vi "Helper SubVI - Filtered Square Wave.vi"(5 "offset":dbl, 7 "reset signal":bool, 9 "duty cycle (%)":dbl=50.0 format="%#.6g", 10 "signal amplitude":dbl=1.0, 11 "frequency":dbl=5.0) -> (0 "error out":errorcluster, 3 "Filtered Square Wave":waveform(dbl))   [LabVIEW 2020]
doc: "Generates a filtered square waveform to be used with the Signal Processing > Waveform Measurements examples."
uses:
  <vilib>/Analysis/3filter.llb/Inverse Chebyshev Filter (DBL).vi
  <vilib>/Analysis/3filter.llb/FIR Filter (DBL).vi
  <vilib>/measure/NI_MABase.lvlib
  <vilib>/Analysis/NI_AALBase.lvlib
panel:
  # "Generates a filtered square waveform to be used with the Signal Processing > Waveform Measurements examples."
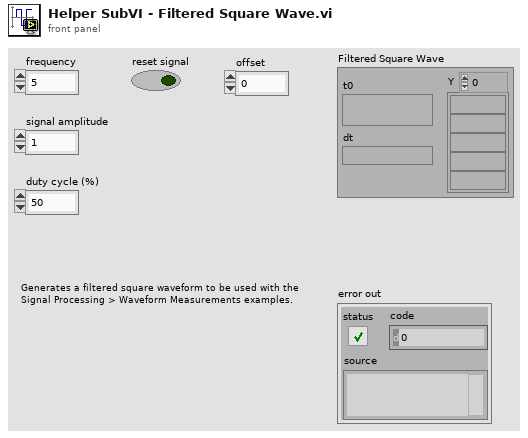
[diagram p1: front panel]
types:
  T1 = enum16{"Sine Wave", "Triangle Wave", "Square Wave", "Sawtooth Wave"}
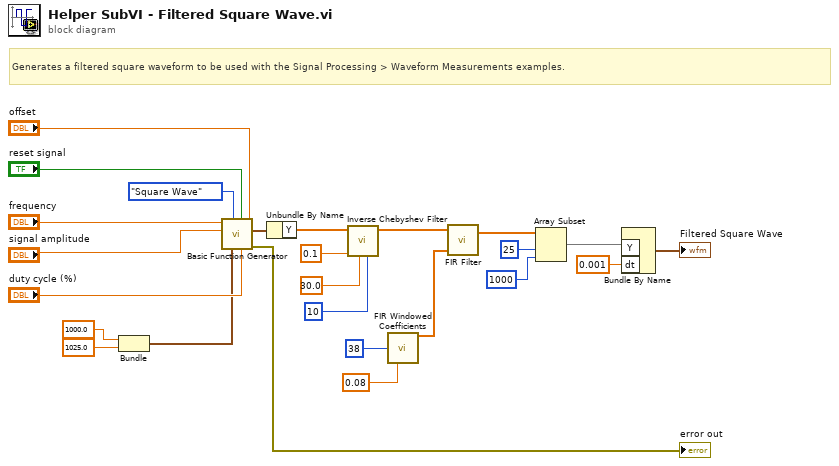
[diagram p0: block diagram]
diagram:
  # "Generates a filtered square waveform to be used with the Signal Processing > Waveform Measurements examples."
  n1 = Bundle("Fs"=1000.0, "Fs"=1025.0) -> (w13:cluster{"Fs":dbl, "Fs":dbl})  [unwired: 1 in]
  n2 = call <vilib>:"Basic Function Generator.vi"("offset"="offset", "square wave duty cycle (%)"="duty cycle (%)", "reset signal"="reset signal", "sampling info"=w13, "signal type"=T1."Square Wave", "amplitude"="signal amplitude", "frequency"="frequency") -> ("error out"=→"error out":errorcluster, "signal out"=w17:waveform(dbl))  [unwired: 2 in, 1 out]
  n3 = Unbundle By Name(w17) -> ("Y"=w16:dbl[])
  n4 = call-poly <vilib>:"Inverse Chebyshev Filter.vi"("order"=10, "attenuation (dB)"=30.0, "low cutoff freq: fl"=0.1, "X"=w16) -> ("Filtered X"=w19:dbl[])  [unwired: 6 in, 1 out]
  n5 = call <vilib>:"FIR Windowed Coefficients.vi"("taps"=38 ("order"), "low cutoff freq: fl"=0.08) -> ("FIR Windowed Coefficients"=w18:dbl[])  [unwired: 12 in, 1 out]
  n6 = call-poly <vilib>:"FIR Filter.vi"("FIR Coefficients"=w18, "X"=w19) -> ("Filtered X"=w12:dbl[])  [unwired: 2 in, 1 out]
  n7 = Array Subset(array=w12, index=25, length=1000) -> (w5:dbl[])
  n8 = Bundle By Name("Y"=w5, "dt"=0.001) -> (→"Filtered Square Wave":waveform(dbl))  [unwired: 1 in]
